vi "Find ProjItem Ref by Path.vi"(8 "error in (no error)":errorcluster, 9 "Path":path, 11 "Proj Ref In":refnum<vi>) -> (0 "error out":errorcluster, 1 "ProjectItem Refnum":refnum<vi>, 3 "Proj Ref Out":refnum<vi>)   [LabVIEW 2018]
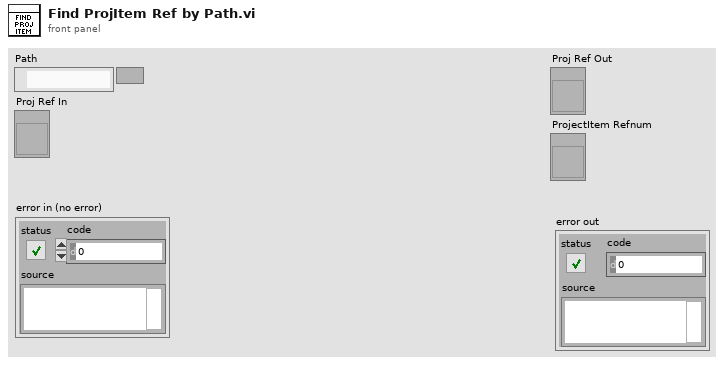
[diagram p1: front panel]
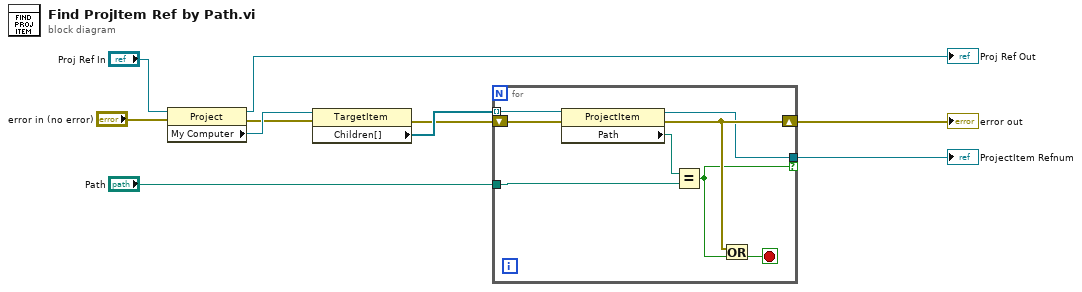
[diagram p0: block diagram]
diagram:
  n1 = property class="Project"(reference="Proj Ref In", error in="error in (no error)") -> (reference out=→"Proj Ref Out":refnum<vi>, error out=w8:errorcluster, "My Computer"=w10:refnum<vi>)
  n2 = property class="TargetItem"(reference=w10, error in=w8) -> (error out=w7:errorcluster, "Children[]"=w9:refnum<vi>[])  [unwired: 1 out]
  n3 = for {
    tunnel: w9 -> [w18] mode=indexing
    shift-right: [w14] -> w3
    shift-left: w7 -> [w17]
    tunnel: "Path" -> [w16]
    tunnel: [w12] -> w2 if=w11
    stop <- w15 stop-if-true
    n4 = property class="ProjectItem"(reference=w18, error in=w17) -> (reference out=w12:refnum<vi>, error out=w14:errorcluster, "Path"=w13:path)
    n5 = Equal?(x=w13, y=w16) -> (x = y?=w11:bool)
    n6 = Or(x=w14, y=w11) -> (x .or. y?=w15:bool)
  }
  "ProjectItem Refnum" <- w2
  "error out" <- w3
